vi "Get Subpanel Ref.vi"(8 "error in":errorcluster, 10 "subpanel UID":i32, 11 "VI info in":T1) -> (0 "error out":errorcluster, 1 "found?":bool, 2 "subpanel ref":refnum<vi>, 3 "VI info out":T1)   [LabVIEW 2010, in "NI_SE_Config Front Panel Layout.lvlib"]
uses:
  NI_SE_Config Front Panel Layout.lvlib
  VI Info.ctl
  VI Panel Layout/VI Panel Layout.lvclass
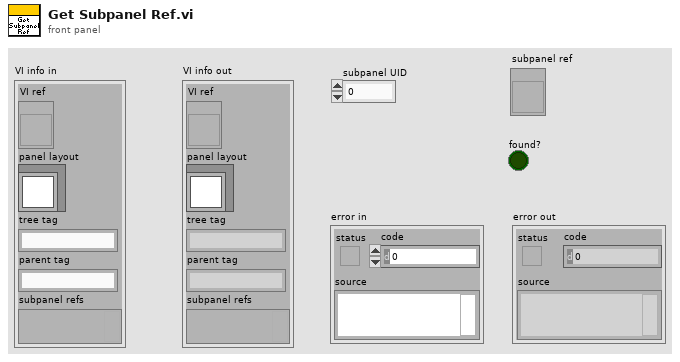
[diagram p1: front panel]
types:
  T1 = typedef "NI_SE_Config Front Panel Layout.lvlib/VI Info.ctl" = cluster{"VI ref":refnum<vi>, "panel layout":refnum<class "VI Panel Layout.lvclass">, "tree tag":string, "parent tag":string, "subpanel refs":variant}
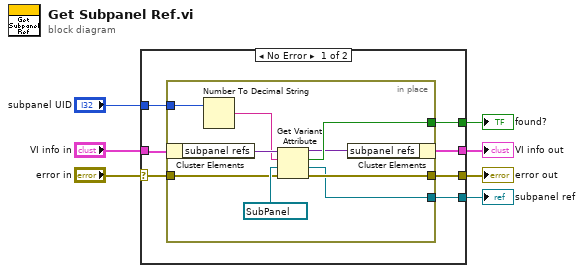
[diagram p0: block diagram]
diagram:
  n1 = case shown="No Error" "error in" {
    selector: "error in" -> [w12 w25]
    tunnel: "VI info in" -> [w14 w24]
    tunnel: [w11 w25] -> w5
    tunnel: [w10 w24] -> w4
    tunnel: "subpanel UID" -> [w13 _]
    tunnel: [w9 _] -> w2
    tunnel: [w8 _] -> w1
    frame No Error {
      n2 = in-place {
        in-place-border: w13 -> [w22]
        in-place-border: w12 -> [w19]
        in-place-border: [w18] -> w11
        in-place-border: [w17] -> w9
        in-place-border: [w16] -> w8
        n3 = in-place-cluster #1(w14) -> ("subpanel refs"=w23:variant)
        n4 = Number To Decimal String(number=w22) -> (decimal integer string=w21:string)  [unwired: 1 in]
        n5 = Get Variant Attribute(Variant=w23, name=w21, default value (empty Variant)=refnum<vi> refnum ("subpanel ref"), error in=w19) -> (duplicate Variant=w15:variant, found=w16:bool, value=w17:refnum<vi>, error out=w18:errorcluster)
        n6 = in-place-cluster #1("subpanel refs"=w15) -> (w10:T1)
      }
    }
    frame Error {
    }
  }
  "VI info out" <- w4
  "error out" <- w5
  "subpanel ref" <- w2
  "found?" <- w1
